vi "Add Record.vi"(8 "Error In (no error)":errorcluster, 10 "Expenses Tracker Record":refnum<class "Expenses Tracker Record.lvclass">[](array[class]), 11 "Database Interactions In":refnum<class "Database Interactions.lvclass">) -> (0 "Error Out":errorcluster, 3 "Database Interactions Out":refnum<class "Database Interactions.lvclass">)   [LabVIEW 2023, in "Database Interactions.lvclass"]
uses:
  Database Interactions.lvclass
  DB Records/Expenses Tracker Record/Expenses Tracker Record.lvclass
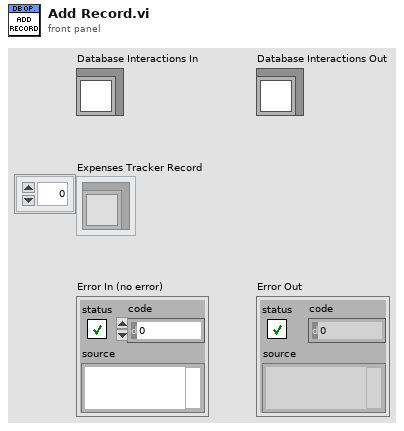
[diagram p1: front panel]
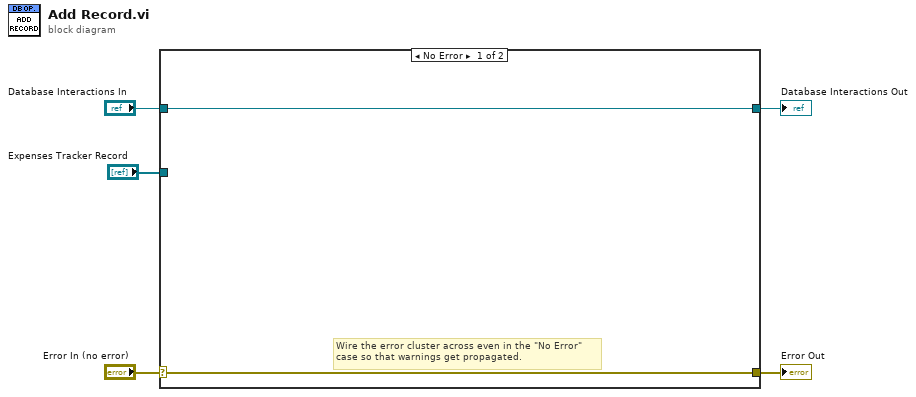
[diagram p0: block diagram]
diagram:
  n1 = case shown="No Error" "Error In (no error)" {
    selector: "Error In (no error)" -> [w6 w9]
    tunnel: [w6 w9] -> w4
    tunnel: [w7 w8] -> w2
    tunnel: "Database Interactions In" -> [w7 w8]
    tunnel: "Expenses Tracker Record" -> [_ _]
    frame No Error {
      # "Wire the error cluster across even in the \"No Error\"\ncase so that warnings get propagated."
    }
    frame Error {
    }
  }
  "Error Out" <- w4
  "Database Interactions Out" <- w2
